vi "TEST Launch from Main.vi"() -> ()   [LabVIEW 2011]
panel:
  out "VIs in memory":string[](array[string])
  in  "Launch":bool
  in  "stop":bool
  in  "Reentrant VI path":path=path "Spawned VI (reentrant).vi"
  # "In this example, launching the asynchronous independent VI  will load the it into memory and run it.\n\nThe asychronous independent VI will manage its own lifetime and leave memory when it finishes execution."
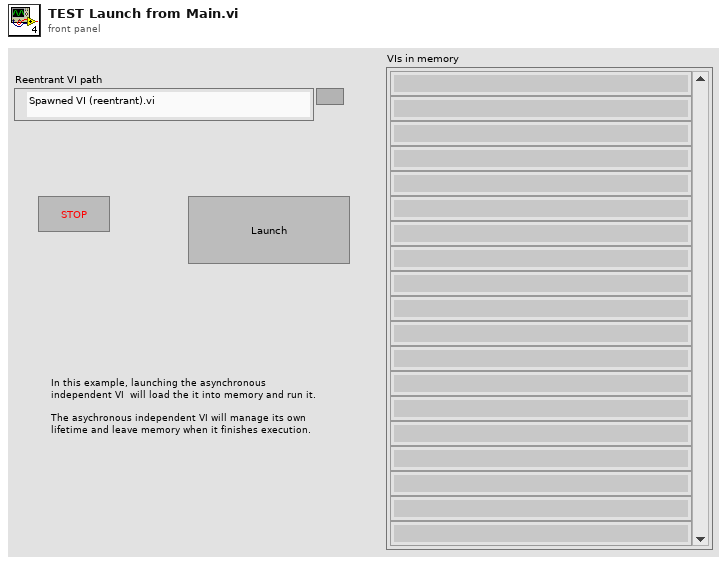
[diagram p1: front panel]
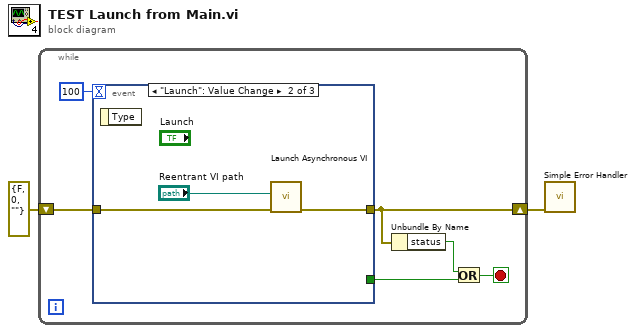
[diagram p0: block diagram]
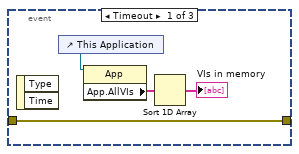
[diagram p2: hidden frame]
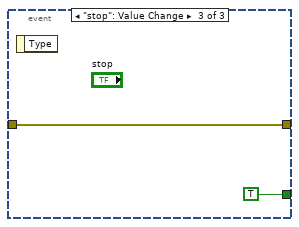
[diagram p3: hidden frame]
diagram:
  n1 = while {
    shift-right: [w5] -> w2
    shift-left: errorcluster {"status"=FALSE, "code"=0, "source"=""} ("error out") -> [w3]
    stop <- w6 stop-if-true
    n2 = event shown="[1] \"Launch\": Value Change" {
      selector: _ -> [_ _ _]
      dyn-events: _ -> [_ _ _]
      timeout: 100 -> [_ _ _]
      tunnel: [w9 w14 w16] -> w5
      tunnel: [_ _ TRUE ("stop")] -> w4
      tunnel: w3 -> [w9 w13 w16]
      event Timeout {
        n3 = event-data() -> ()  [unwired: 1 in, 2 out]
        n4 = control-ref of="This Application"() -> (w12:refnum<vi>)
        n5 = property class="App"(reference=w12) -> ("App.AllVIs"=w10:string[])  [unwired: 1 in, 2 out]
        n6 = Sort 1D Array(array=w10) -> (sorted array=→"VIs in memory":string[])
      }
      event "Launch": Value Change {
        n7 = event-data() -> ()  [unwired: 1 in, 1 out]
        n8 = call "Launch Asynchronous VI.vi"("error in (no error)"=w13, "VI path"="Reentrant VI path") -> ("error out"=w14:errorcluster)  [unwired: 9 in]
      }
      event "stop": Value Change {
        n9 = event-data() -> ()  [unwired: 1 in, 1 out]
      }
    }
    n10 = Unbundle By Name(w5) -> ("status"=w7:bool)
    n11 = Or(x=w7, y=w4) -> (x .or. y?=w6:bool)
  }
  n12 = call <vilib>:"Simple Error Handler.vi"("error in (no error)"=w2) -> ()  [unwired: 4 in, 5 out]
